vi "Get and Set FP Status.vi"(8 "错误输入（无错误）":errorcluster, 9 "Mode":enum16{"Read", "Write"}(ring), 10 "前面板窗口:状态":T1(ring), 11 "VI Ref In":refnum<vi>) -> (0 "错误输出":errorcluster, 3 "FP.State":T1(ring))   [LabVIEW 2012, in "VIRef.lvlib"]
uses:
  VIRef.lvlib
panel:
  out "VI Ref Out":refnum<vi>
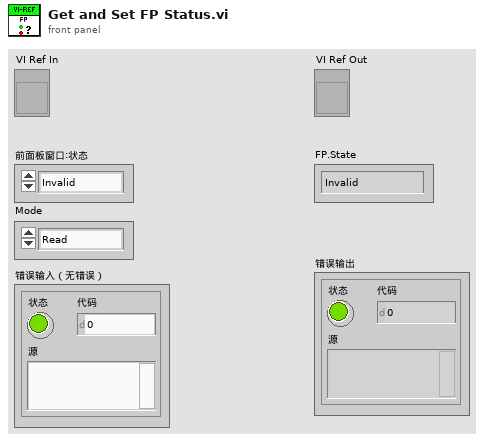
[diagram p1: front panel]
types:
  T1 = enum32{"Invalid", "Standard", "Closed", "Hidden", "Minimized", "Maximized"}
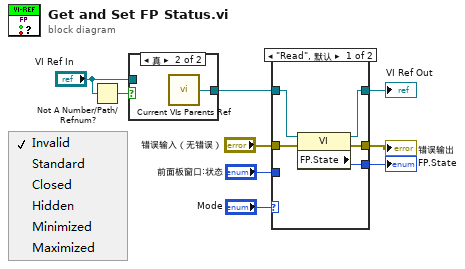
[diagram p0: block diagram]
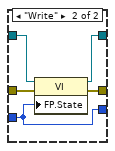
[diagram p2: hidden frame]
diagram:
  n1 = Not A Number/Path/Refnum?(number/path/refnum="VI Ref In") -> (NaN/Path/Refnum?=w8:bool)
  n2 = case shown="真" w8 {
    tunnel: [w10 w11] -> w4
    tunnel: "VI Ref In" -> [w10 _]
    frame False {
    }
    frame True {
      n3 = call "Current VIs Parents Ref.vi"() -> ("Calling VI's Reference"=w11:refnum<vi>)  [unwired: 2 in]
    }
  }
  n4 = case shown="\"Read\", 默认" "Mode" {
    tunnel: "错误输入（无错误）" -> [w14 w21]
    tunnel: [w13 w20] -> w6
    tunnel: w4 -> [w16 w17]
    tunnel: [w15 w18] -> w3
    tunnel: [w12 w19] -> w2
    tunnel: "前面板窗口:状态" -> [_ w19]
    frame "Read", Default {
      n5 = property class="VI"(reference=w16, error in=w14) -> (reference out=w15:refnum<vi>, error out=w13:errorcluster, "FP.State"=w12:T1)
    }
    frame "Write" {
      n6 = property class="VI"(reference=w17, error in=w21, "FP.State"=w19) -> (reference out=w18:refnum<vi>, error out=w20:errorcluster)
    }
  }
  "VI Ref Out" <- w3
  "错误输出" <- w6
  "FP.State" <- w2
